vi "Channels.vi"(8 "error in (no error)":errorcluster, 11 "Group in":refnum<class "Group Config.lvclass">) -> (0 "error out":errorcluster, 2 "Channels":refnum<class "Channel Config.lvclass">[](array[class]), 3 "Group out":refnum<class "Group Config.lvclass">)   [LabVIEW 2020, in "VolatusConfig.lvlib" / "Group Config.lvclass"]
uses:
  Group Config.lvclass
  C:/dev/lv20CE/relink/lv-volatus/VolatusConfig/VolatusConfigElement/VolatusConfigElement.lvclass
  Channel/Channel Config.lvclass
  Meta Type.ctl
  VolatusConfigElement/VolatusConfigElement.lvclass/VolatusConfigElement.ctl
  VolatusConfigElement/Element.vi
  lv-cdm/CDM-Config/Config Lookup/Match Meta.vi
  lv-cdm/CDM-Config/Config Element/Owner.vi
  lv-cdm/CDM-Config/Config Manager/Lookup Descendant.vi
  lv-cdm/CDM-Config/Config Filter/Config Lookup.lvclass
  Group Config.lvclass/Group Config.ctl
  VolatusConfig.lvlib
  VolatusConfigElement/VolatusConfigElement.lvclass
  C:/dev/lv20CE/relink/lv-volatus/VolatusConfig/Group/Group Config.lvclass
  C:/dev/lv20CE/relink/lv-volatus/VolatusConfig/Channel/Channel Config.lvclass
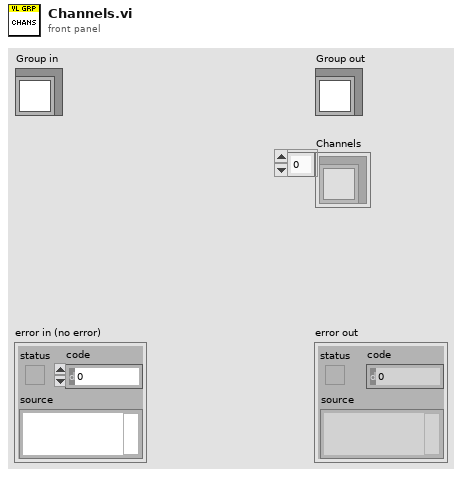
[diagram p1: front panel]
types:
  T1 = typedef "VolatusConfig.lvlib/Meta Type.ctl" = enum16{"UNKNOWN", "VL_System", "VL_Cluster", "VL_Node", "VL_Task", "VL_Group", "VL_Channel", "VL_Task_List", "VL_Scaling", "VL_Sensor", "VL_Sensor_List", "VL_Scale"}
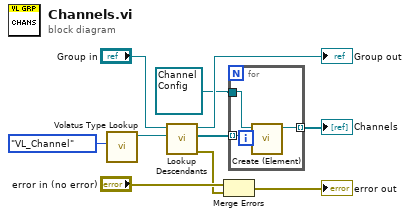
[diagram p0: block diagram]
diagram:
  n1 = call "Volatus Type Lookup.vi"("Meta Type"=Meta_Type."VL_Channel") -> ("Config Lookup out"=w8:refnum<class "Config Lookup.lvclass">)  [unwired: 9 in, 1 out]
  n2 = call "Lookup Descendants.vi"("Lookup"=w8, "VolatusConfigElement in"="Group in") -> ("error out"=w4:errorcluster, "Descendants"=w7:refnum<class "Config Element.lvclass">[], "VolatusConfigElement out"=→"Group out":refnum<class "Group Config.lvclass">)  [unwired: 7 in]
  n3 = Merge Errors("error in (no error)", w4) -> (→"error out":errorcluster)
  n4 = for {
    tunnel: w7 -> [w12] mode=indexing
    tunnel: [w13] -> w6 mode=indexing
    tunnel: refnum<class "Channel Config.lvclass"> refnum ("VolatusConfig.lvlib:Channel.lvclass") -> [w11]
    n5 = call "Create (Element).vi"("Element"=w12, "VolatusConfigElement in"=w11) -> ("VolatusConfigElement out"=w13:refnum<class "Channel Config.lvclass">)  [unwired: 8 in, 1 out]
  }
  "Channels" <- w6
